vi "ConvertBandUnit.vi"(7 "Amplitude Scale":T1(ring), 8 "error in (no error)":errorcluster, 9 "Desired Unit":string, 10 "Channel Properties":variant, 11 "EU RMS":sgl) -> (0 "error out":errorcluster, 3 "Scaled Value":sgl)   [LabVIEW 2017]
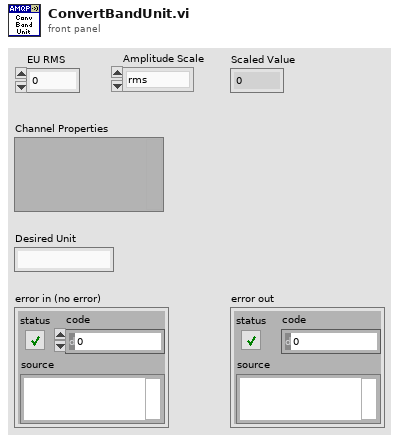
[diagram p1: front panel]
types:
  T1 = enum16{"rms", "peak", "pk-pk", "phase", "<none>"}
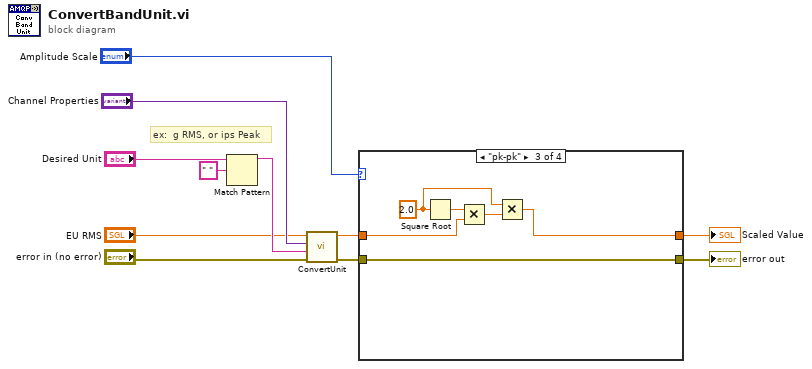
[diagram p0: block diagram]
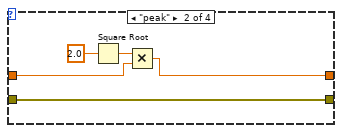
[diagram p3: hidden frame]
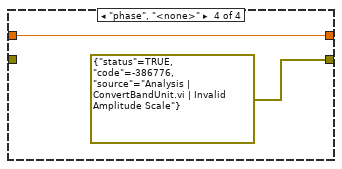
[diagram p4: hidden frame]
diagram:
  # "ex:  g RMS, or ips Peak"
  n1 = Match Pattern(string="Desired Unit", regular expression=" ") -> (before substring=w8:string)  [unwired: 1 in, 3 out]
  n2 = call <vilib>:"ConvertUnit.vi"("error in"="error in (no error)", "Desired Unit"=w8, "Channel Properties"="Channel Properties", "Value"="EU RMS") -> ("error out"=w3:errorcluster, "Scaled Value"=w11:sgl)  [unwired: 6 in]
  n3 = case shown="\"pk-pk\"" "Amplitude Scale" {
    tunnel: [w13 w14 w22 errorcluster {"status"=TRUE, "code"=-386776, "source"="Analysis | ConvertBandUnit.vi | Invalid Amplitude Scale"} ("error in (no error)")] -> w9
    tunnel: w3 -> [w13 w14 w22 _]
    tunnel: [w12 w15 w19 w26] -> w10
    tunnel: w11 -> [w12 w16 w23 w26]
    frame "rms" {
    }
    frame "peak" {
      n4 = Square Root(x=sgl 2.0) -> (sqrt(x)=w17:sgl)
      n5 = Multiply(x=w17, y=w16) -> (x*y=w15:sgl)
    }
    frame "pk-pk" {
      w20 = sgl 2.0 ("x")
      n6 = Square Root(x=w20) -> (sqrt(x)=w24:sgl)
      n7 = Multiply(x=w24, y=w23) -> (x*y=w21:sgl)
      n8 = Multiply(x=w20, y=w21) -> (x*y=w19:sgl)
    }
    frame "phase", "<none>" {
    }
  }
  "Scaled Value" <- w10
  "error out" <- w9
